vi "GetParamWavePrbsType.vi"(3 "error in (no error)":errorcluster, 4 "ParamWave Name":string, 5 "VISA resource name":refnum<visa-resource-name>) -> (0 "error out":errorcluster, 1 "Prbs Type":u16(ring) items=[" PRBS-7", " PRBS-9", " PRBS-11", " PRBS-15", " PRBS-23", " PRBS-31"], 2 "VISA resource name out":refnum<visa-resource-name>)   [LabVIEW 2020, in "Active Technologies AWG3000.lvlib"]
uses:
  Active Technologies AWG3000.lvlib
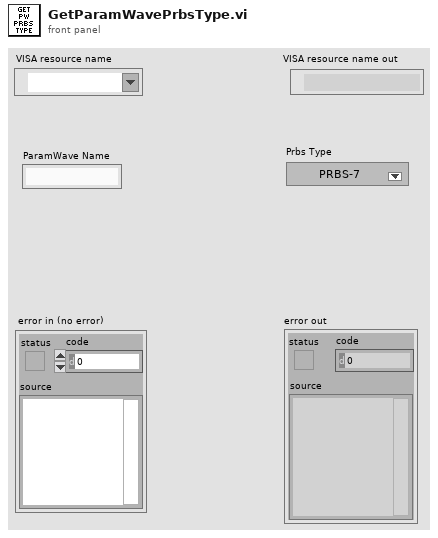
[diagram p1: front panel]
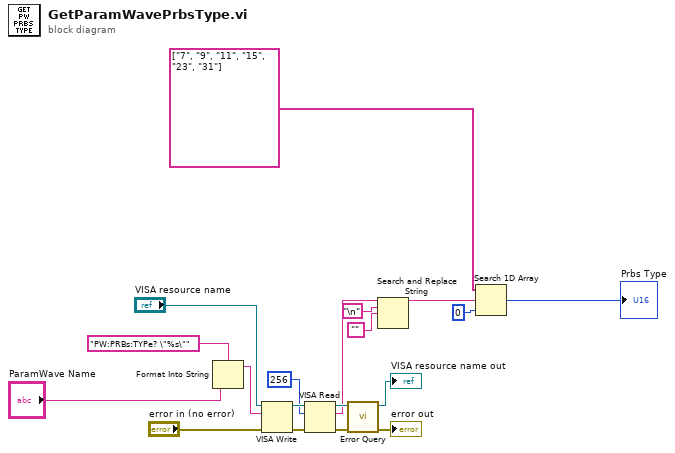
[diagram p0: block diagram]
diagram:
  n1 = Format Into String(format string="PW:PRBs:TYPe? \"%s\"" ("write buffer"), "ParamWave Name") -> (resulting string=w9:string)  [unwired: 2 in, 1 out]
  n2 = VISA Write(VISA resource name="VISA resource name", write buffer=w9, error in (no error)="error in (no error)") -> (VISA resource name out=w16:refnum<visa-resource-name>, error out=w15:errorcluster)  [unwired: 1 out]
  n3 = VISA Read(VISA resource name=w16, byte count=u32 256, error in (no error)=w15) -> (VISA resource name out=w13:refnum<visa-resource-name>, read buffer=w4:string, error out=w12:errorcluster)  [unwired: 1 out]
  n4 = call "Error Query.vi"("error in (no error)"=w12, "VISA resource name"=w13) -> ("error out"=→"error out":errorcluster, "VISA resource name out"=→"VISA resource name out":refnum<visa-resource-name>)  [unwired: 6 in, 2 out]
  n5 = Search and Replace String(input string=w4, search string="\n", replace string="") -> (result string=w5:string)  [unwired: 5 in, 3 out]
  n6 = Search 1D Array(1D array=string[] ["7", "9", "11", "15", "23", "31"], element=w5, start index (0)=0) -> (index of element=→"Prbs Type":i32)
